vi "ParamsArray2BinFile.vi"(7 "Default params as\nData type const":T1={"TaskIDs"={"DAQ tasks"={"Px taskID"=0, "Py taskID"=0, "Pz taskID"=0, "AOM taskID"=0, "Clock taskID"=0, "AI taskID"=0}, "DVEHandle"=refnum}, "Manual Control"={"Rotation Control"={"Phase"=0.0, "A amp (0-120)"=75.0, "B amp (0-120)"=53.3, "mean freq  [MHz]\ndefault 39.99"=40.0, "freq difference [Hz]"=2.0, "Enable A"=TRUE, "Enable B"=TRUE}, "X piezo\n [nm]"=0.0, "Y peizo\n [nm]"=0.0, "trap height\n [nm]"=5.012658227848101, "AOM0 \nPower"=0.2}, "Piezo Calibr"={"Px2Vx(AO)"=nan, "Py2Vy(AO)"=nan, "Pz2Vz(AO)"=nan, "Min Px"=nan, "Min Py"=nan, "Min Pz"=nan, "Max Px"=nan, "Max Py"=nan, "Max Pz"=nan, "Vx0 (V)"=nan, "Vy0 (V)"=nan, "Vz0 (V)"=nan}, "Instrument Calibr"={"Angular compensation coeffs"=[], "TetherCenter"={"TrapX_AO 0 [nm]"=nan, "TrapY_AO 0 [nm]"=nan, "TrapZ_AO 0 [nm]"=nan}, "XYZsignal baseline"={"Xsignal0"=nan, "Ysignal0"=nan, "Zsignal0"=nan, "Zsig slope"=nan, "Z bead0"=nan}, "S and P to Vs0"={"Vs0/P"=1.0, "Vs0/S"=1.0}, "Psi"=0.0, "ePS:eRL drift correlation"={"Interc P"=nan, "Slope P"=nan, "Interc S"=nan, "Slope S"=nan}, "Current piezo volt AO"={"Vpx_AO [V]"=nan, "Vpy_AO [V]"=nan, "Vpz_AO [V]"=nan}}, "Cylinder Calibr"={"ZStiff"=nan, "Zsens"=nan, "AngStiff"=nan, "XStiff"=nan, "Xsens"=nan, "MaxEllip"=nan, "YStiff"=nan, "Ysens"=nan, "FocalShift"=nan, "Sfz"=nan, "1/Sz"=nan, "Stau"=nan, "Sfx"=nan, "1/Sx"=nan, "1/Sang"=nan, "Sfy"=nan, "1/Sy"=nan, "1/focal"=nan, "ZsignalHeightDependence (1/nm)"=0.0}, "DAQParams"={"Buffer size"=nan, "Scanning rate"=nan, "Average"=nan, "Sampling rate"=nan, "set dt"=nan}, "DAQ channel offsets"={"A0 [V]"=0.0, "D0 [V]"=0.0, "P0  [V]"=0.0, "S0 [V]"=0.0, "L0 [V]"=0.0, "R0 [V]"=0.0, "Vpx0 [V]"=0.0, "Vpy0 [V]"=0.0, "Vpz0 [V]"=0.0, "Vsum0 [V]"=0.0, "Vpx_AO0 [V]"=0.0, "Vpy_AO0 [V]"=0.0, "Vpz_AO0 [V]"=0.0}, "Z bead polynomial coeffs"=[nan, nan, nan, nan], "Skip button ref"=refnum, "z bead lookup table"={"z signal"=[], "z bead"=[]}, "SP->power Matrix"=[], "Ms2p"=[], "Mp2s"=[], "Polynomial coeff V_px,y,z 2 position (nm)"=[]} {"Cylinder Calibr"."ZsignalHeightDependence (1/nm)" format="%.4e"; "Instrument Calibr"."Psi" format="%#_2f"; "Manual Control"."Y peizo\n [nm]" step=100.0 scale=0.0..30000.0; "Manual Control"."AOM0 \nPower" scale=0.0..1.0; "Manual Control"."X piezo\n [nm]" step=100.0 scale=0.0..30000.0; "Manual Control"."Rotation Control"."mean freq  [MHz]\ndefault 39.99" min=0.0 step=0.01; "Manual Control"."Rotation Control"."B amp (0-120)" min=0.0 max=120.0 step=0.1 format="%.1f"; "Manual Control"."Rotation Control"."A amp (0-120)" min=0.0 max=120.0 step=0.1 format="%.1f"; "Manual Control"."Rotation Control"."Phase" scale=0.0..360.0; "Manual Control"."trap height\n [nm]" scale=1000.0..7500.0; "TaskIDs"."DAQ tasks"."Px taskID" format="%x"; "TaskIDs"."DAQ tasks"."Py taskID" format="%x"; "TaskIDs"."DAQ tasks"."Pz taskID" format="%x"; "TaskIDs"."DAQ tasks"."AOM taskID" format="%x"; "TaskIDs"."DAQ tasks"."Clock taskID" format="%x"; "TaskIDs"."DAQ tasks"."AI taskID" format="%x"}, 8 "error in":errorcluster, 9 "write (0) or read (1)":i32(ring)=1 items=["Write", "Read"], 10 "file path in":path, 11 "Array of Params in":T1[](array[typedef]) {"Cylinder Calibr"."ZsignalHeightDependence (1/nm)" format="%.4e"; "Instrument Calibr"."Psi" format="%#_2f"; "Manual Control"."Y peizo\n [nm]" step=100.0 scale=0.0..30000.0; "Manual Control"."AOM0 \nPower" scale=0.0..1.0; "Manual Control"."X piezo\n [nm]" step=100.0 scale=0.0..30000.0; "Manual Control"."Rotation Control"."mean freq  [MHz]\ndefault 39.99" min=0.0 step=0.01; "Manual Control"."Rotation Control"."B amp (0-120)" min=0.0 max=120.0 step=0.1 format="%.1f"; "Manual Control"."Rotation Control"."A amp (0-120)" min=0.0 max=120.0 step=0.1 format="%.1f"; "Manual Control"."Rotation Control"."Phase" scale=0.0..360.0; "Manual Control"."trap height\n [nm]" scale=1000.0..7500.0; "TaskIDs"."DAQ tasks"."Px taskID" format="%x"; "TaskIDs"."DAQ tasks"."Py taskID" format="%x"; "TaskIDs"."DAQ tasks"."Pz taskID" format="%x"; "TaskIDs"."DAQ tasks"."AOM taskID" format="%x"; "TaskIDs"."DAQ tasks"."Clock taskID" format="%x"; "TaskIDs"."DAQ tasks"."AI taskID" format="%x"}) -> (0 "error out":errorcluster, 1 "Good?":bool, 2 "file path out":path, 3 "Array of Params out":T1[](array[typedef]) {"Cylinder Calibr"."ZsignalHeightDependence (1/nm)" format="%.4e"; "Instrument Calibr"."Psi" format="%#_2f"; "Manual Control"."Y peizo\n [nm]" step=100.0 scale=0.0..30000.0; "Manual Control"."AOM0 \nPower" scale=0.0..1.0; "Manual Control"."X piezo\n [nm]" step=100.0 scale=0.0..30000.0; "Manual Control"."Rotation Control"."mean freq  [MHz]\ndefault 39.99" min=0.0 step=0.01; "Manual Control"."Rotation Control"."B amp (0-120)" min=0.0 max=120.0 step=0.1 format="%.1f"; "Manual Control"."Rotation Control"."A amp (0-120)" min=0.0 max=120.0 step=0.1 format="%.1f"; "Manual Control"."Rotation Control"."Phase" scale=0.0..360.0; "Manual Control"."trap height\n [nm]" scale=1000.0..7500.0; "TaskIDs"."DAQ tasks"."Px taskID" format="%x"; "TaskIDs"."DAQ tasks"."Py taskID" format="%x"; "TaskIDs"."DAQ tasks"."Pz taskID" format="%x"; "TaskIDs"."DAQ tasks"."AOM taskID" format="%x"; "TaskIDs"."DAQ tasks"."Clock taskID" format="%x"; "TaskIDs"."DAQ tasks"."AI taskID" format="%x"})   [LabVIEW 2020, in "Initialization.lvlib" / "FileManagement.lvlib"]
uses:
  FileManagement.lvlib
  Param.ctl
  ManualCtrl.ctl
  DVESetting.ctl
  CylinderCalibrNew.ctl
  SignalConversion/DAQChannelOffsets.ctl
  <vilib>/Analysis/Matrix/Datatypes/RealMatrix.ctl
  Initialization.lvlib
  <vilib>/Analysis/Matrix/NI_Matrix.lvlib
  SignalConversion/SignalConverson.lvlib
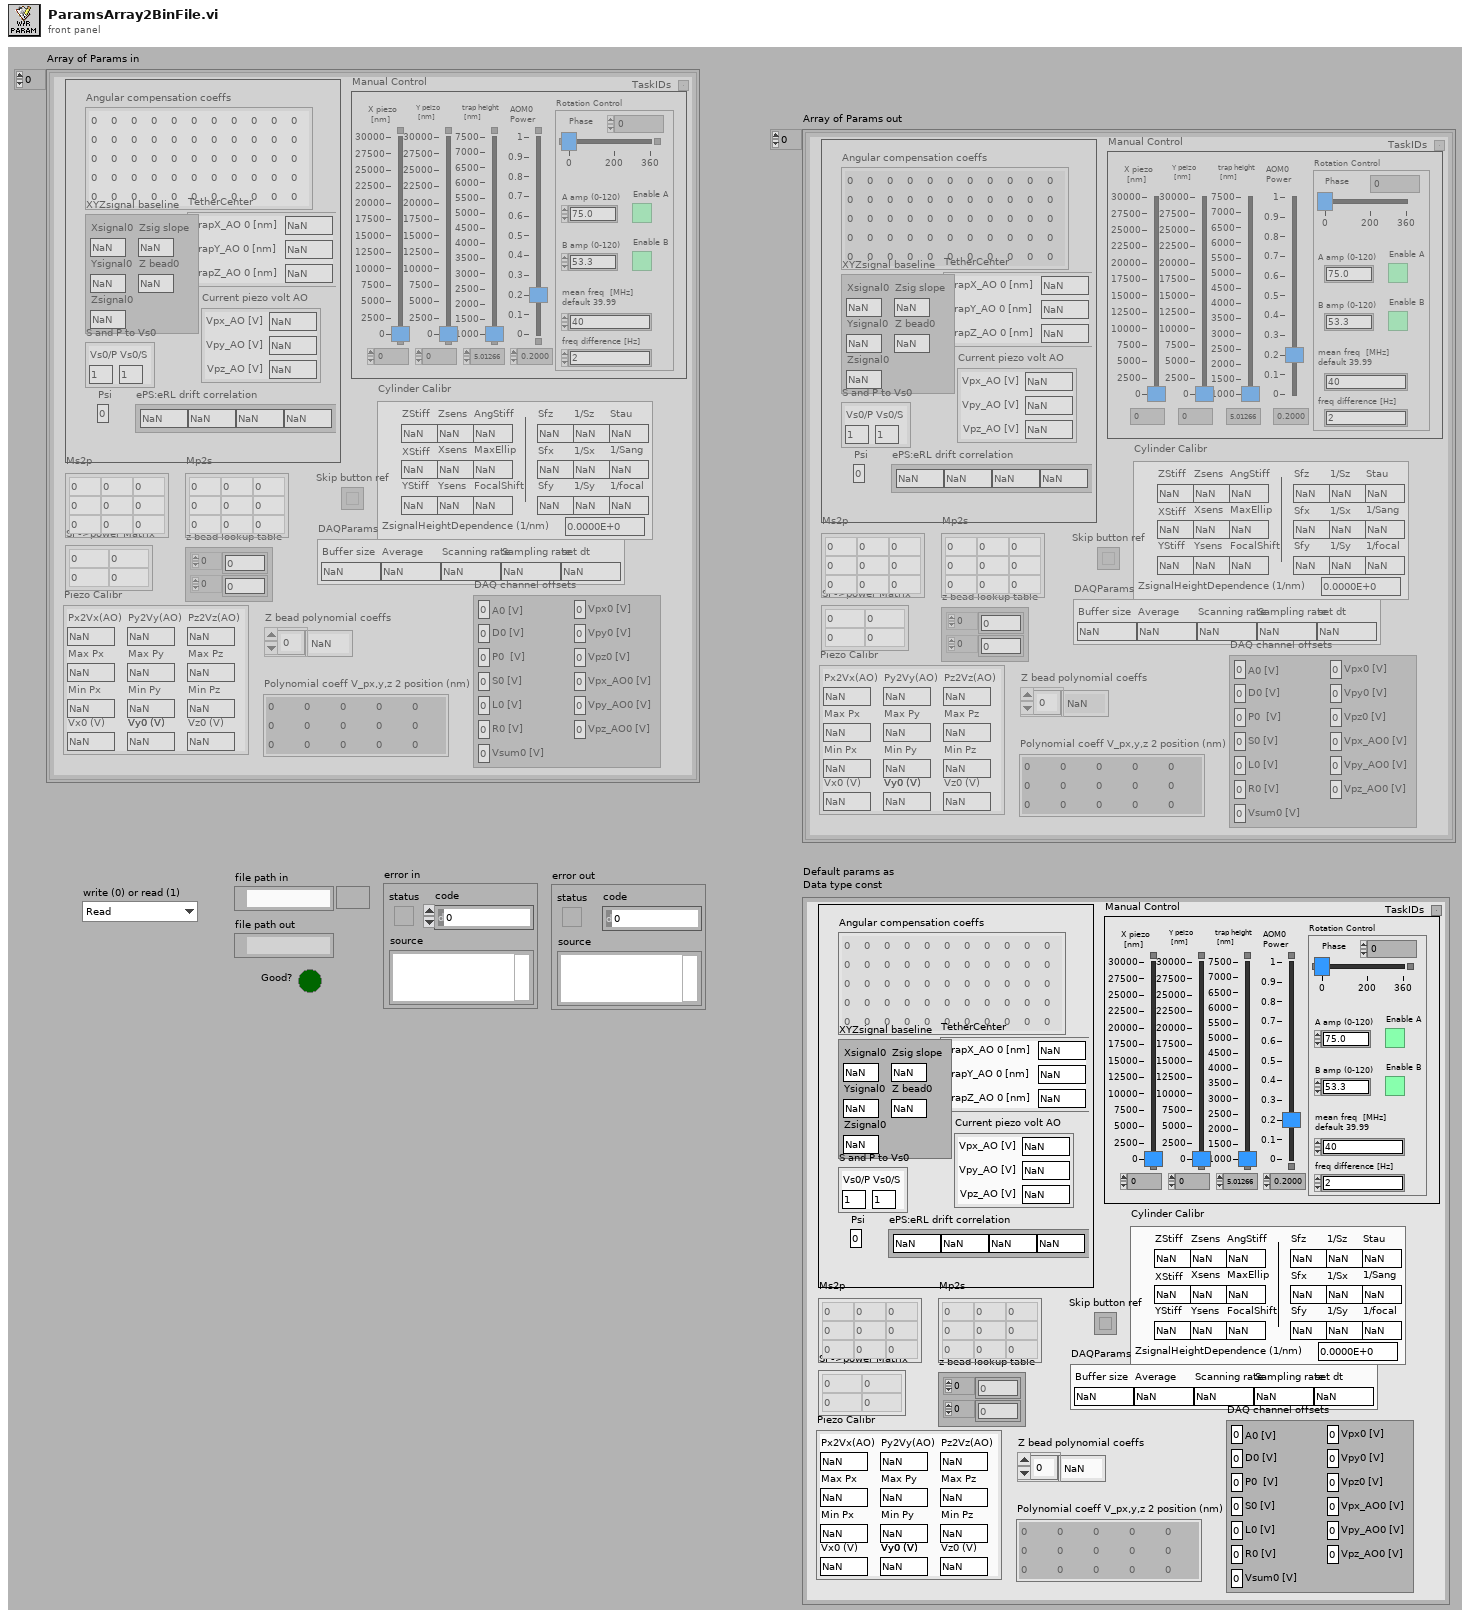
[diagram p1: front panel]
types:
  T1 = typedef "Initialization.lvlib/Param.ctl" = cluster{"TaskIDs":cluster{"DAQ tasks":cluster{"Px taskID":u32, "Py taskID":u32, "Pz taskID":u32, "AOM taskID":u32, "Clock taskID":u32, "AI taskID":u32}, "DVEHandle":refnum<file>}, "Manual Control":T2, "Piezo Calibr":cluster{"Px2Vx(AO)":dbl, "Py2Vy(AO)":dbl, "Pz2Vz(AO)":dbl, "Min Px":dbl, "Min Py":dbl, "Min Pz":dbl, "Max Px":dbl, "Max Py":dbl, "Max Pz":dbl, "Vx0 (V)":dbl, "Vy0 (V)":dbl, "Vz0 (V)":dbl}, "Instrument Calibr":cluster{"Angular compensation coeffs":dbl[][], "TetherCenter":cluster{"TrapX_AO 0 [nm]":dbl, "TrapY_AO 0 [nm]":dbl, "TrapZ_AO 0 [nm]":dbl}, "XYZsignal baseline":cluster{"Xsignal0":dbl, "Ysignal0":dbl, "Zsignal0":dbl, "Zsig slope":dbl, "Z bead0":dbl}, "S and P to Vs0":cluster{"Vs0/P":dbl, "Vs0/S":dbl}, "Psi":dbl, "ePS:eRL drift correlation":cluster{"Interc P":dbl, "Slope P":dbl, "Interc S":dbl, "Slope S":dbl}, "Current piezo volt AO":cluster{"Vpx_AO [V]":dbl, "Vpy_AO [V]":dbl, "Vpz_AO [V]":dbl}}, "Cylinder Calibr":T4, "DAQParams":cluster{"Buffer size":dbl, "Scanning rate":dbl, "Average":dbl, "Sampling rate":dbl, "set dt":dbl}, "DAQ channel offsets":T5, "Z bead polynomial coeffs":dbl[], "Skip button ref":refnum<vi>, "z bead lookup table":cluster{"z signal":dbl[], "z bead":dbl[]}, "SP->power Matrix":T6, "Ms2p":T6, "Mp2s":T6, "Polynomial coeff V_px,y,z 2 position (nm)":dbl[][]}
  T2 = typedef "Initialization.lvlib/ManualCtrl.ctl" = cluster{"Rotation Control":T3, "X piezo\n [nm]":dbl, "Y peizo\n [nm]":dbl, "trap height\n [nm]":dbl, "AOM0 \nPower":dbl}
  T3 = typedef "Initialization.lvlib/DVESetting.ctl" = cluster{"Phase":dbl, "A amp (0-120)":dbl, "B amp (0-120)":dbl, "mean freq  [MHz]\ndefault 39.99":dbl, "freq difference [Hz]":dbl, "Enable A":bool, "Enable B":bool}
  T4 = typedef "Initialization.lvlib/CylinderCalibrNew.ctl" = cluster{"ZStiff":dbl, "Zsens":dbl, "AngStiff":dbl, "XStiff":dbl, "Xsens":dbl, "MaxEllip":dbl, "YStiff":dbl, "Ysens":dbl, "FocalShift":dbl, "Sfz":dbl, "1/Sz":dbl, "Stau":dbl, "Sfx":dbl, "1/Sx":dbl, "1/Sang":dbl, "Sfy":dbl, "1/Sy":dbl, "1/focal":dbl, "ZsignalHeightDependence (1/nm)":dbl}
  T5 = typedef "SignalConverson.lvlib/DAQChannelOffsets.ctl" = cluster{"A0 [V]":dbl, "D0 [V]":dbl, "P0  [V]":dbl, "S0 [V]":dbl, "L0 [V]":dbl, "R0 [V]":dbl, "Vpx0 [V]":dbl, "Vpy0 [V]":dbl, "Vpz0 [V]":dbl, "Vsum0 [V]":dbl, "Vpx_AO0 [V]":dbl, "Vpy_AO0 [V]":dbl, "Vpz_AO0 [V]":dbl}
  T6 = typedef "NI_Matrix.lvlib/RealMatrix.ctl" = dbl[][]
  T7 = enum16{"open", "replace", "create", "open or create", "replace or create", "replace or create with confirmation"}
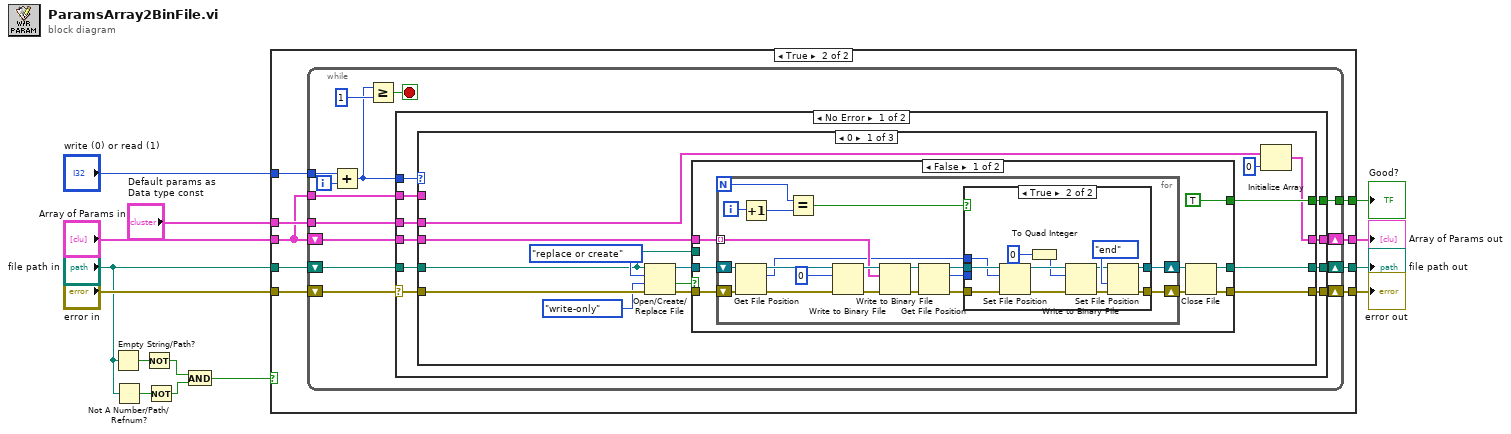
[diagram p0: block diagram]
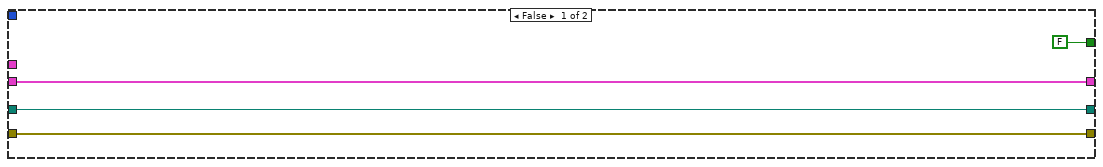
[diagram p2: hidden frame]
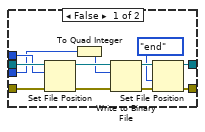
[diagram p3: hidden frame]
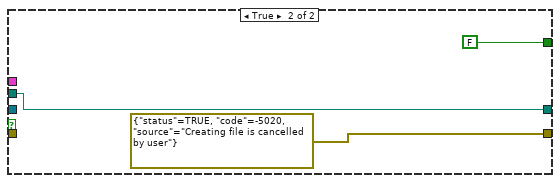
[diagram p4: hidden frame]
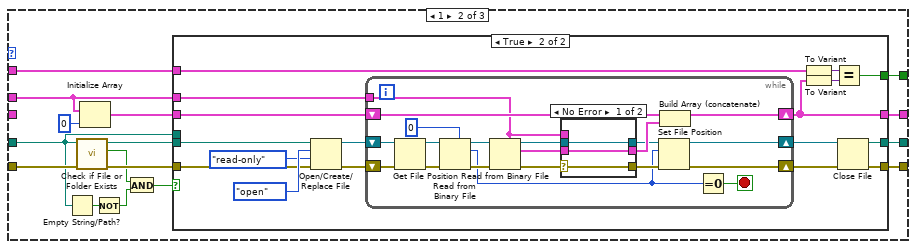
[diagram p5: hidden frame]
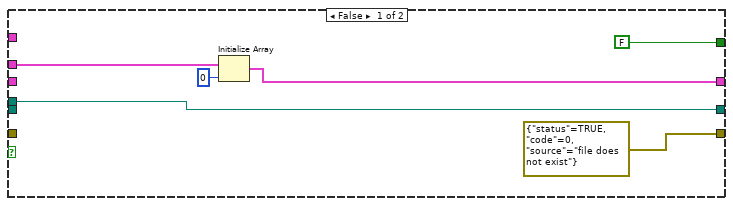
[diagram p6: hidden frame]
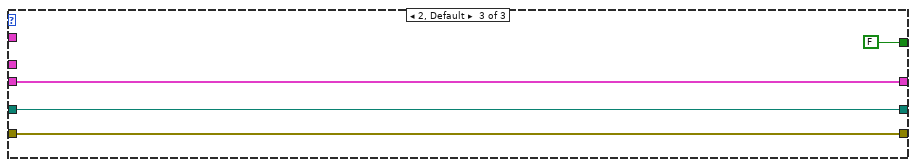
[diagram p8: hidden frame]
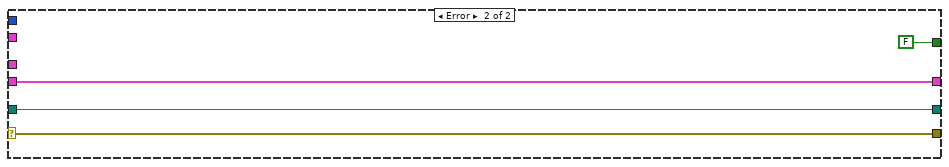
[diagram p9: hidden frame]
diagram:
  n1 = Empty String/Path?(string/path="file path in") -> (empty?=w6:bool)
  n2 = Not A Number/Path/Refnum?(number/path/refnum="file path in") -> (NaN/Path/Refnum?=w3:bool)
  n3 = Not(x=w6) -> (.not. x?=w5:bool)
  n4 = Not(x=w3) -> (.not. x?=w4:bool)
  n5 = And(x=w5, y=w4) -> (x .and. y?=w1:bool)
  n6 = case shown="True" w1 {
    tunnel: [w16 w27] -> w14
    tunnel: [w17 w26] -> w13
    tunnel: [w18 w25] -> w12
    tunnel: "error in" -> [w16 w24]
    tunnel: [FALSE w23] -> w10
    tunnel: "write (0) or read (1)" -> [_ w22]
    tunnel: "Default params as\nData type const" -> [_ w21]
    tunnel: "Array of Params in" -> [w18 w20]
    tunnel: "file path in" -> [w17 w19]
    frame False {
    }
    frame True {
      n7 = while {
        shift-right: [w39] -> w27
        shift-left: w24 -> [w33]
        shift-right: [w38] -> w26
        shift-left: w19 -> [w41]
        shift-right: [w37] -> w25
        shift-left: w20 -> [w40]
        tunnel: w21 -> [w36]
        tunnel: w20 -> [w35]
        tunnel: [w34] -> w23
        tunnel: w22 -> [w31]
        i -> [w32]
        stop <- w29 stop-if-true
        n8 = Add(x=w31, y=w32) -> (x+y=w28:i32)
        n9 = Greater Or Equal?(x=w28, y=1) -> (x >= y?=w29:bool)
        n10 = case shown="No Error" w33 {
          selector: w33 -> [w42 w192]
          tunnel: w41 -> [w51 w191]
          tunnel: w40 -> [w50 w190]
          tunnel: [w49 w192] -> w39
          tunnel: [w48 w191] -> w38
          tunnel: w28 -> [w47 _]
          tunnel: [w46 w190] -> w37
          tunnel: w36 -> [w45 _]
          tunnel: w35 -> [w44 _]
          tunnel: [w43 FALSE] -> w34
          frame No Error {
            n11 = case shown="0" w47 {
              tunnel: w51 -> [w55 w125 w188]
              tunnel: w42 -> [w65 w127 w187]
              tunnel: w50 -> [w61 _ w186]
              tunnel: [w54 w132 w187] -> w49
              tunnel: [w53 w133 w188] -> w48
              tunnel: [w56 w136 w186] -> w46
              tunnel: w45 -> [w57 w129 _]
              tunnel: w44 -> [_ w135 _]
              tunnel: [w59 w134 FALSE] -> w43
              frame 0 {
                n12 = Open/Create/Replace File(file path (use dialog)=w55, error in=w65, operation (0:open)=T7."replace or create", access (0:read/write)=enum16{"read/write", "read-only", "write-only"}."write-only") -> (refnum out=w63:refnum<file>, cancelled=w52:bool, error out=w62:errorcluster)  [unwired: 2 in]
                n13 = case shown="False" w52 {
                  tunnel: w63 -> [w73 _]
                  tunnel: w62 -> [w72 _]
                  tunnel: w61 -> [w71 _]
                  tunnel: [TRUE FALSE] -> w59
                  tunnel: w55 -> [_ w118]
                  tunnel: [w67 errorcluster {"status"=TRUE, "code"=-5020, "source"="Creating file is cancelled by user"} ("error out")] -> w54
                  tunnel: [w66 w118] -> w53
                  frame False {
                    n14 = for {
                      N -> [w75]
                      tunnel: w71 -> [w80] mode=indexing
                      shift-right: [w79] -> w68
                      shift-left: w73 -> [w92]
                      shift-right: [w88] -> w69
                      shift-left: w72 -> [w93]
                      i -> [w77]
                      n15 = Get File Position(4:w93, 7:w92) -> (0:w89:errorcluster, 2:w78:i64, 3:w90:refnum<file>)
                      n16 = Increment(x=w77) -> (x+1=w76:i32)
                      n17 = Equal?(x=w75, y=w76) -> (x = y?=w74:bool)
                      n18 = Write to Binary File(file (use dialog)=w90, data=i64 0, error in=w89) -> (refnum out=w84:refnum<file>, error out=w81:errorcluster)  [unwired: 3 in, 1 out]
                      n19 = Write to Binary File(file (use dialog)=w84, data=w80, error in=w81) -> (refnum out=w83:refnum<file>, error out=w82:errorcluster)  [unwired: 3 in, 1 out]
                      n20 = Get File Position(4:w82, 7:w83) -> (0:w87:errorcluster, 2:w85:i64, 3:w86:refnum<file>)
                      n21 = case shown="True" w74 {
                        tunnel: w87 -> [w96 w111]
                        tunnel: [w100 w110] -> w88
                        tunnel: w86 -> [w103 w112]
                        tunnel: w78 -> [w98 w108]
                        tunnel: w85 -> [w97 _]
                        tunnel: [w95 w109] -> w79
                        frame False {
                          n22 = Set File Position(offset (in bytes) (0)=w98, refnum=w103, error in=w96) -> (refnum out=w104:refnum<file>, error out=w105:errorcluster)  [unwired: 1 in]
                          n23 = To Quad Integer(1:w97) -> (0:w94:i64)
                          n24 = Write to Binary File(file (use dialog)=w104, data=w94, error in=w105) -> (refnum out=w102:refnum<file>, error out=w101:errorcluster)  [unwired: 3 in, 1 out]
                          n25 = Set File Position(refnum=w102, from (0:start)=enum16{"start", "end", "current"}."end", error in=w101) -> (refnum out=w95:refnum<file>, error out=w100:errorcluster)  [unwired: 1 in]
                        }
                        frame True {
                          n26 = Set File Position(offset (in bytes) (0)=w108, refnum=w112, error in=w111) -> (refnum out=w114:refnum<file>, error out=w113:errorcluster)  [unwired: 1 in]
                          n27 = To Quad Integer(1:i64 0) -> (0:w106:i64)
                          n28 = Write to Binary File(file (use dialog)=w114, data=w106, error in=w113) -> (refnum out=w115:refnum<file>, error out=w116:errorcluster)  [unwired: 3 in, 1 out]
                          n29 = Set File Position(refnum=w115, from (0:start)=enum16{"start", "end", "current"}."end", error in=w116) -> (refnum out=w109:refnum<file>, error out=w110:errorcluster)  [unwired: 1 in]
                        }
                      }
                    }
                    n30 = Close File(refnum=w68, error in=w69) -> (path=w66:path, error out=w67:errorcluster)
                  }
                  frame True {
                  }
                }
                n31 = Initialize Array(w57, 0 ("dimension size")) -> (w56:T1[])
              }
              frame 1 {
                n32 = Empty String/Path?(string/path=w125) -> (empty?=w124:bool)
                n33 = call <vilib>:"Check if File or Folder Exists.vi"("error in (no error)"=w127, "path"=w125) -> ("error out"=w126:errorcluster, "file or folder exists?"=w122:bool, "dup path"=w128:path)  [unwired: 7 in]
                n34 = Initialize Array(w129, 0 ("dimension size")) -> (w130:T1[])
                n35 = Not(x=w124) -> (.not. x?=w123:bool)
                n36 = And(x=w122, y=w123) -> (x .and. y?=w121:bool)
                n37 = case shown="True" w121 {
                  tunnel: [w140 w155] -> w136
                  tunnel: w129 -> [w141 w159]
                  tunnel: [w137 w150] -> w133
                  tunnel: [errorcluster {"status"=TRUE, "code"=0, "source"="file does not exist"} ("error out") w151] -> w132
                  tunnel: w130 -> [_ w158]
                  tunnel: w135 -> [_ w154]
                  tunnel: [FALSE w153] -> w134
                  tunnel: w125 -> [w137 _]
                  tunnel: w128 -> [_ w144]
                  tunnel: w126 -> [_ w143]
                  frame False {
                    n38 = Initialize Array(w141, 0 ("dimension size")) -> (w140:T1[])
                  }
                  frame True {
                    n39 = Open/Create/Replace File(file path (use dialog)=w144, error in=w143, operation (0:open)=T7."open", access (0:read/write)=enum16{"read/write", "read-only", "write-only"}."read-only") -> (refnum out=w145:refnum<file>, error out=w146:errorcluster)  [unwired: 2 in, 1 out]
                    n40 = while {
                      shift-right: [w178] -> w155
                      shift-left: w158 -> [w176]
                      tunnel: w159 -> [w161]
                      shift-right: [w165] -> w149
                      shift-left: w145 -> [w170]
                      shift-right: [w164] -> w152
                      shift-left: w146 -> [w173]
                      stop <- w179 stop-if-true
                      n41 = Get File Position(4:w173, 7:w170) -> (0:w172:errorcluster, 3:w171:refnum<file>)  [unwired: 1 out]
                      n42 = Read from Binary File(5:i64 0, 8:w172, 11:w171) -> (0:w174:errorcluster, 2:w160:i64, 3:w175:refnum<file>)  [unwired: 3 in, 1 out]
                      n43 = Read from Binary File(5:w161, 8:w174, 11:w175) -> (0:w168:errorcluster, 2:w167:T1, 3:w169:refnum<file>)  [unwired: 3 in, 1 out]
                      n44 = case shown="No Error" w168 {
                        selector: w168 -> [w181 _]
                        tunnel: w169 -> [w180 w183]
                        tunnel: w167 -> [w182 _]
                        tunnel: [w182 w184] -> w166
                        tunnel: [w181 _] -> w163
                        tunnel: [w180 w183] -> w162
                        tunnel: w161 -> [_ w184]
                        frame No Error {
                        }
                        frame Error {
                        }
                      }
                      n45 = Set File Position(offset (in bytes) (0)=w160, refnum=w162, error in=w163) -> (refnum out=w165:refnum<file>, error out=w164:errorcluster)  [unwired: 1 in]
                      n46 = Build Array (concatenate)(w176, w166) -> (w178:T1[])
                      n47 = Equal To 0?(x=w160) -> (x = 0?=w179:bool)
                    }
                    n48 = To Variant(anything=w154) -> (Variant=w157:variant)
                    n49 = To Variant(anything=w155) -> (Variant=w156:variant)
                    n50 = Equal?(x=w157, y=w156) -> (x = y?=w153:bool)
                    n51 = Close File(refnum=w149, error in=w152) -> (path=w150:path, error out=w151:errorcluster)
                  }
                }
              }
              frame 2, Default {
              }
            }
          }
          frame Error {
          }
        }
      }
    }
  }
  "error out" <- w14
  "file path out" <- w13
  "Array of Params out" <- w12
  "Good?" <- w10
